vi "执行流程.vi"(8 "error in (no error)":errorcluster caption="错误输入（无错误）", 11 "零件加工流程 输入":refnum<class "零件加工流程.lvclass"> caption="DNL_LabVIEW Object in") -> (0 "error out":errorcluster caption="错误输出", 3 "零件加工流程 输出":refnum<class "零件加工流程.lvclass"> caption="DNL_LabVIEW Object out")   [LabVIEW 2013, in "零件加工流程.lvclass"]
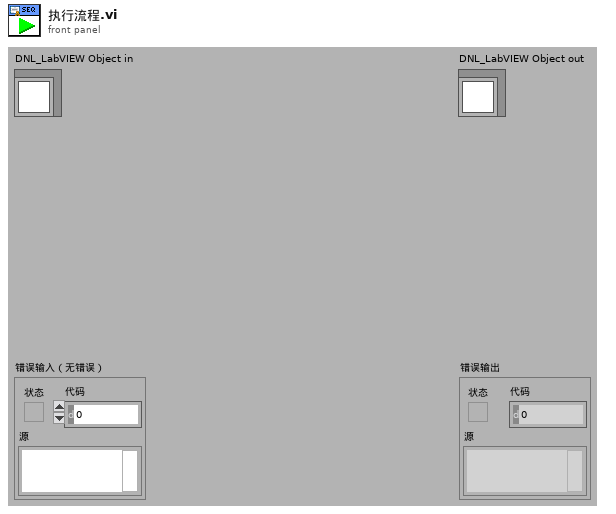
[diagram p1: front panel]
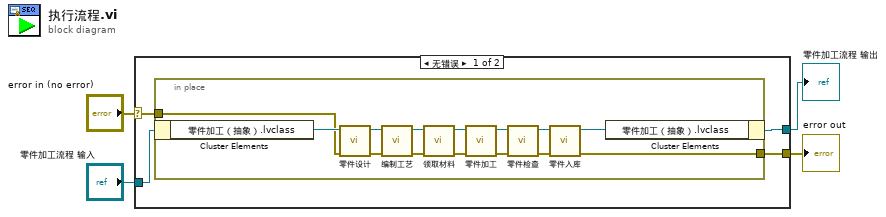
[diagram p0: block diagram]
diagram:
  n1 = case shown="无错误" "error in (no error)" {
    selector: "error in (no error)" -> [w7 w24]
    tunnel: [w6 w24] -> w3
    tunnel: [w5 w23] -> w1
    tunnel: "零件加工流程 输入" -> [w8 w23]
    frame No Error {
      n2 = in-place {
        in-place-border: w7 -> [w10]
        in-place-border: [w9] -> w6
        n3 = in-place-cluster #1(w8) -> ("零件加工（抽象）.lvclass"=w22:refnum<class "零件加工（抽象）.lvclass">)
        n4 = call-dynamic "零件设计.vi"("error in (no error)"=w10, "零件加工（抽象） 输入"=w22) -> ("error out"=w16:errorcluster, "零件加工（抽象） 输出"=w21:refnum<class "零件加工（抽象）.lvclass">)  [unwired: 7 in, 1 out]
        n5 = call-dynamic "编制工艺.vi"("error in (no error)"=w16, "零件加工（抽象） 输入"=w21) -> ("error out"=w15:errorcluster, "零件加工（抽象） 输出"=w20:refnum<class "零件加工（抽象）.lvclass">)  [unwired: 7 in, 1 out]
        n6 = call-dynamic "领取材料.vi"("error in (no error)"=w15, "零件加工（抽象） 输入"=w20) -> ("error out"=w14:errorcluster, "零件加工（抽象） 输出"=w19:refnum<class "零件加工（抽象）.lvclass">)  [unwired: 7 in, 1 out]
        n7 = call-dynamic "零件加工.vi"("error in (no error)"=w14, "零件加工（抽象） 输入"=w19) -> ("error out"=w13:errorcluster, "零件加工（抽象） 输出"=w18:refnum<class "零件加工（抽象）.lvclass">)  [unwired: 7 in, 1 out]
        n8 = call-dynamic "零件检查.vi"("error in (no error)"=w13, "零件加工（抽象） 输入"=w18) -> ("error out"=w12:errorcluster, "零件加工（抽象） 输出"=w17:refnum<class "零件加工（抽象）.lvclass">)  [unwired: 7 in, 1 out]
        n9 = call-dynamic "零件入库.vi"("error in (no error)"=w12, "零件加工（抽象） 输入"=w17) -> ("error out"=w9:errorcluster, "零件加工（抽象） 输出"=w11:refnum<class "零件加工（抽象）.lvclass">)  [unwired: 7 in, 1 out]
        n10 = in-place-cluster #1("零件加工（抽象）.lvclass"=w11) -> (w5:refnum<class "零件加工流程.lvclass">)
      }
    }
    frame Error {
    }
  }
  "error out" <- w3
  "零件加工流程 输出" <- w1
